vi "Do Command.vi"(6 "Actions In":refnum<class "Iteration Actions.lvclass">, 7 "Variables in":refnum<class "Variables.lvclass">, 8 "error in (no error)":errorcluster, 9 "Sequence Time":T1, 10 "VolatusAPI":refnum<class "VolatusAPI.lvclass">, 11 "Numeric Command in":refnum<class "Numeric Command.lvclass">) -> (0 "error out":errorcluster, 4 "Actions":refnum<class "Iteration Actions.lvclass">, 5 "Variables":refnum<class "Variables.lvclass">)   [LabVIEW 2020, in "VolatusSeq.lvlib" / "Numeric Command.lvclass"]
uses:
  Numeric Command.lvclass
  Variables/Variables.lvclass
  Volatus/VolatusAPI/VolatusAPI.lvclass
  Iteration Actions/Iteration Actions.lvclass
  Numeric Command.lvclass/Numeric Command.ctl
  Iteration Actions/Iteration Actions.lvclass/Iteration Actions.ctl
  Sequence Time.ctl
  VolatusSeq.lvlib
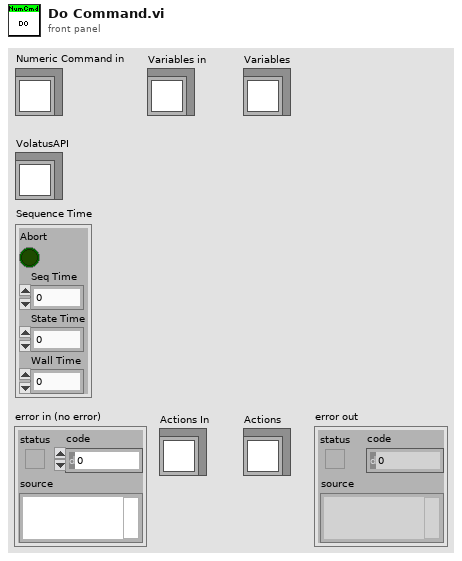
[diagram p1: front panel]
types:
  T1 = typedef "VolatusSeq.lvlib/Sequence Time.ctl" = cluster{"Abort":bool, "Seq Time":dbl, "State Time":dbl, "Wall Time":dbl}
  T2 = typedef "CmdAnalog.lvlib/Data.ctl" = cluster{"channel":string, "value":dbl}
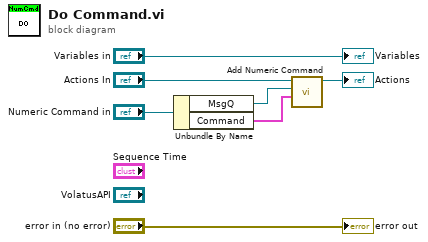
[diagram p0: block diagram]
diagram:
  n1 = Unbundle By Name("Numeric Command in") -> ("MsgQ"=w2:refnum<class "MessageQ.lvclass">, "Command"=w1:T2)
  n2 = call "Add Numeric Command.vi"("CmdAnalog"=w1, "MsgQ"=w2, "Iteration Actions in"="Actions In") -> ("Iteration Actions out"=→"Actions":refnum<class "Iteration Actions.lvclass">)  [unwired: 7 in, 1 out]
  "error out" <- "error in (no error)"
  "Variables" <- "Variables in"
